vi "Dashboard Main.vi"() -> ()   [LabVIEW 2015]
uses:
  <vilib>/Utility/miscctls.llb/LVRowAndColumnTypeDef.ctl
  <vilib>/event_ctls.llb/eventvkey.ctl
  <vilib>/Rock Robotics/WPI/Dashboard/WPI_DashboardLogging Global.vi
  <vilib>/Rock Robotics/Network Tables/NT Read Numeric Array.vi
  <vilib>/Rock Robotics/Network Tables/NT Read Boolean.vi
  <vilib>/Rock Robotics/Network Tables/NT Write Boolean.vi
  <vilib>/Utility/config.llb/Write Key (String).vi
  <vilib>/Utility/config.llb/Write Key (I32).vi
  <vilib>/Utility/config.llb/NI_LVConfig.lvlib
panel:
  in  "TCP":refnum<k5>
  in  "Rec Mode":enum32{"Stop", "Record", "Playback"}(radio)
  in  "Vision":u16(ring) items=["Camera Off", "USB Camera SW", "USB Camera HW", "IP Camera"]
  out "Camera IP":string
  out "Image Message":string="Timeout in Camera Communications"
  in  "Dashboard Tab":T1(tab)
  in  "Select Auto":string(combo)
  out "NT Connection":bool
  in  "Camera Settings":T2={"Frame Rate"=30, "Compression"=30, "Size"=1} {"Frame Rate" scale=1.0..30.0; "Size" items=["640x480", "320x240", "160x120"]}
  out "MotorChart R":cluster{"Numeric":dbl, "Numeric":dbl}(graph)
  out "MotorChart L":T3(graph)
  out "MotorSliders R":cluster{"MotorSlide1":dbl, "MotorSlide2":dbl} {"MotorSlide2" scale=-1.0..1.0 scale format="%#_2e"; "MotorSlide1" scale=-1.0..1.0 scale format="%#_2e"}
  out "MotorSliders L":T4 {"MotorSlide4 2" scale=0.0..14.0 scale format="%#_2e"; "MotorSlide2" scale=-1.0..1.0 scale format="%#_2e"; "MotorSlide1" scale=-1.0..1.0 scale format="%#_2e"}
  out "Gyro":dbl(knob) scale=0.0..360.0
  out "JS1 Z":dbl(slide) scale=-1.0..1.0 scale format="%#_2e"
  out "JS1 Graph":cluster{"X":dbl, "Y":dbl}[](graph)
  out "JS1 Buttons":T5
  out "JS2 Z":dbl(slide) scale=-1.0..1.0 scale format="%#_2e"
  out "JS2 Graph":cluster{"X":dbl, "Y":dbl}[](graph)
  out "JS2 Buttons":T5
  out "Mode":T6(ring)=enum."Auto Disabled"
  in  "DB Camera Config":bool
  out "fps":dbl format="%#.1g"
  out "Mbps":dbl format="%#.1g"
  out "Mbps LED":bool
  in  "DB/String 9":string
  in  "DB/String 8":string
  in  "DB/String 7":string
  in  "DB/String 6":string
  in  "DB/String 5":string
  in  "DB/String 4":string
  in  "DB/String 3":string
  in  "DB/String 2":string
  in  "DB/String 1":string
  in  "DB/String 0":string
  in  "DB/Slider 0":dbl(slide) scale=0.0..5.0
  in  "DB/Slider 1":dbl(slide) scale=0.0..5.0
  in  "DB/Slider 2":dbl(slide) scale=0.0..5.0
  in  "DB/Slider 3":dbl(slide) scale=0.0..5.0
  out "DB/LED 3":bool
  out "DB/LED 2":bool
  out "DB/LED 1":bool
  out "DB/LED 0":bool
  in  "DB/Button 3":bool
  in  "DB/Button 2":bool
  in  "DB/Button 1":bool
  in  "DB/Button 0":bool caption="New Name"
  in  "Lower Shoot On Start of Auto":bool=TRUE
  in  "Auto Mode \nSelector":dbl
  out "?":dbl(slide)=88.0 scale=78.0..98.0
  out "POT Online?":bool
  out "?":dbl(knob)=87.99999517335185 scale=78.0..98.0
  out "True Solid Value":dbl=88.0
  out "POT Sensor":dbl(knob)=88.0000526149156 scale=78.0..98.0
  out "Low Sensor":bool=TRUE
  out "High Sensor":bool=TRUE
  in  "Test Slider":dbl(slide) scale=0.0..100.0 scale format="%#_3g"
  in  "On/Off":bool caption="Solenoid"
  in  "Test Name":u16(ring) items=["Select the test to run..."]
  in  "Test Tree":string(tree)
  in  "Motor":cluster{"Value":dbl, "Enable":bool} {"Value" scale=-1.0..1.0 scale format="%#_3g"}
  out "Progress":T7 {"Test Progress" scale=0.0..100.0}
  in  "Rev/Fwd":cluster{"Forward":bool, "Reverse":bool}
  in  "Test Ring":u16(ring) items=["Monochrome", "Color"]
  out "Cmd Status":string
  in  "Execute Command":bool
  in  "Command Params":string[][](table)
  in  "Command Selection":i32(listbox)
  in  "CheckList":i32(listbox)
  out "Tree":string(tree)
  out "Camera Image":T8(plugin-control)
  out "Background":bool
  # "Left"
  # "Front"
  # "Right"
  # "Battery"
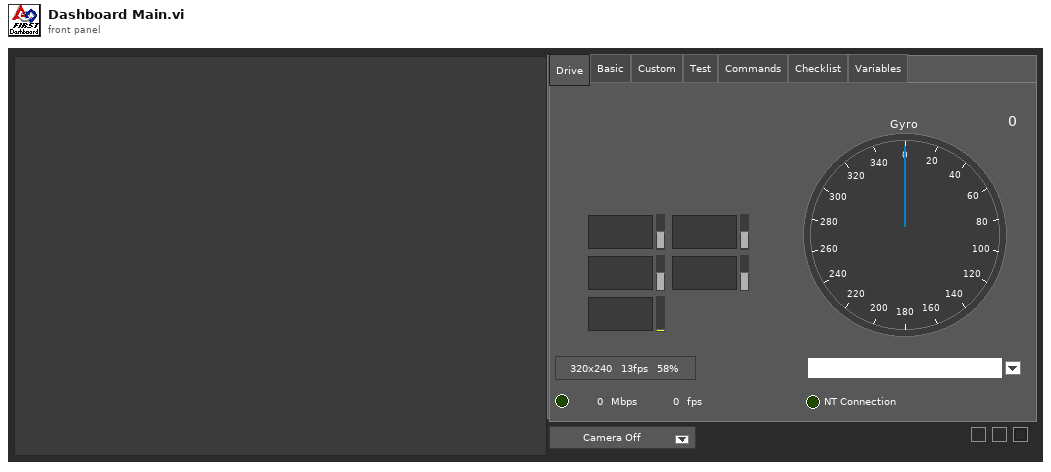
[diagram p1: front panel]
types:
  T1 = enum32{"Drive", "Basic", "Custom", "Test", "Commands", "Checklist", "Variables"}
  T2 = cluster{"Frame Rate":i32, "Compression":i32, "Size":u16}
  T3 = cluster{"Numeric":dbl, "Numeric":dbl, "Battery V":dbl}
  T4 = cluster{"MotorSlide1":dbl, "MotorSlide2":dbl, "MotorSlide4 2":dbl}
  T5 = cluster{bool, bool, bool, bool, bool, bool, bool, bool, bool, bool, bool, bool}
  T6 = enum8{"Tele-Op Disabled", "Tele-Op Enabled", "Auto Disabled", "Auto Enabled", "Test Disabled", "Test Enabled", "Disconnected", "No Code", "E-Stop"}
  T7 = cluster{"Test Progress":u8, "Test Progress Text":string}
  T8 = typedef "IMAQ Image.ctl" = refnum<image>
  T9 = cluster{"IDs":cluster{"RPC field ID":u16, "Unique ID":u16}, "String":string}
  T10 = enum32{"Drive", "Basic", "Custom", "Test", "Checklist", "Variables"}
  T11 = typedef "Image Type" = u32
  T12 = cluster{"Camera Image":refnum<vi>, "Dashboard Tab":refnum<vi>, "Background":refnum<vi>, "Vision":refnum<vi>, "Rec Mode":refnum<vi>, "Test Slider":refnum<vi>, "On/Off ":refnum<vi>, "Test Ring":refnum<vi>, "Rev/Fwd":refnum<vi>, "Test Name":refnum<vi>, "Motor":refnum<vi>, "Progress":refnum<vi>, "CheckList":refnum<vi>, "Tree":refnum<vi>, "Test Tree":refnum<vi>, "Command Params":refnum<vi>, "Command Selection":refnum<vi>, "Execute Command":refnum<vi>, "Cmd Status":refnum<vi>}
  T13 = cluster{"Error Strings":string, "Disable Counts":cluster{u16, u16}, "Rail Faults":cluster{u16, u16, u16}, "Robot IP":string, "DB Mode":u8, "Event Info":cluster{"Name":string, "Type":u8, "Number":u16, "Replay":u8}, "Camera Addr":string}
  T14 = cluster{"Storage":cluster{"Disk Free":u64, "RAM Block":u32, "RAM free":u32}, "CPU Utilization":cluster{"CPU % ISR":sgl, "CPU % Time Crit":sgl, "CPU % Timed Str":sgl, "CPU % High":sgl, "CPU % Above":sgl, "CPU % Normal":sgl, "CPU % Low":sgl}, "CAN":cluster{"% Bus Utilization":sgl, "Bus Off Cnt":u32, "TX_FIFO Full Cnt":u32, "Receive Error Cnt":u8, "Transmit Error Cnt":u8}, "HID":cluster{"HID Outputs":u32, "Rumble Low":u16, "Rumble High":u16}[]}
  T15 = cluster{"Status bits":cluster{"Test Mode":bool, "Autonomous":bool, "Enabled":bool, "Code Start":bool, "Brownout":bool, "Reserved 2":bool, "Reserved 3":bool, "E-Stop":bool}, "Code Trace":cluster{"Disabled":bool, "TeleOp":bool, "Auto":bool, "Test":bool}, "Controller Type":enum16{"unknown", "cRIO", "roboRio"}, "Code?":enum16{"unknown", "noCode", "code"}, "Battery V":dbl}
  T16 = cluster{"Control Bits":cluster{"TestMode":bool, "Autonomous":bool, "Enabled":bool, "FMS Present":bool, bool, bool, bool, "E-Stop":bool}, "Team Station ":u8, "Countdown":sgl, "Joystick Values":cluster{"Axes":dbl[], "Buttons":bool[], "POVs":i16[]}[]}
  T17 = cluster{"Axes":dbl[], "Buttons":bool[], "POVs":i16[]}[]
  T18 = cluster{"Axes":dbl[], "Buttons":bool[], "POVs":i16[]}
  T19 = cluster{"Buttons[0]":bool, "Buttons[1]":bool, "Buttons[2]":bool, "Buttons[3]":bool, "Buttons[4]":bool, "Buttons[5]":bool, "Buttons[6]":bool, "Buttons[7]":bool, "Buttons[8]":bool, "Buttons[9]":bool, "Buttons[10]":bool, "Buttons[11]":bool}
  T20 = typedef "NI_LVConfig.lvlib/Config Data RefNum.ctl" = refnum<k1>
  T21 = cluster{"Operation":enum16{"Update", "Clear"}, "Color Box":u32}[]
  T22 = typedef "eventvkey.ctl" = enum16{"ASCII", "Enter", "Return", "Shift", "Ctrl", "Alt", "Cmd", "Opt", "Caps", "NumLock", "Clear", "Break", "Up", "Down", "Left", "Right", "Insert", "Delete", "Home", "End", "PageUp", "PageDown", "Escape", "Help", "Pause", "ScrollLock", "F1", "F2", "F3", "F4", "F5", "F6", "F7", "F8", "F9", "F10", "F11", "F12", "F13", "F14", "F15", "F16", "F17", "F18", "F19", "F20", "F21", "F22", "F23", "F24", "Play", "VolumeUp", "VolumeDown", "Mute", "Two Byte Char"}
  T23 = cluster{"Image Size":bool, "Image Type":bool, "Pixel Value":bool, "ROI Information":bool, "Zoom Factor":bool}
  T24 = enum8{"Enabled", "Disabled", "Disabled and Grayed Out"}
  T25 = cluster{"Operation":enum16{"Update", "Clear"}, "Color Box":u32}
  T26 = typedef "LVRowAndColumnTypeDef.ctl" = cluster{"Row":i32, "Column":i32}
  T27 = cluster{"Shift":bool, "Ctrl":bool, "Alt":bool, "Cmd":bool, "Opt":bool}
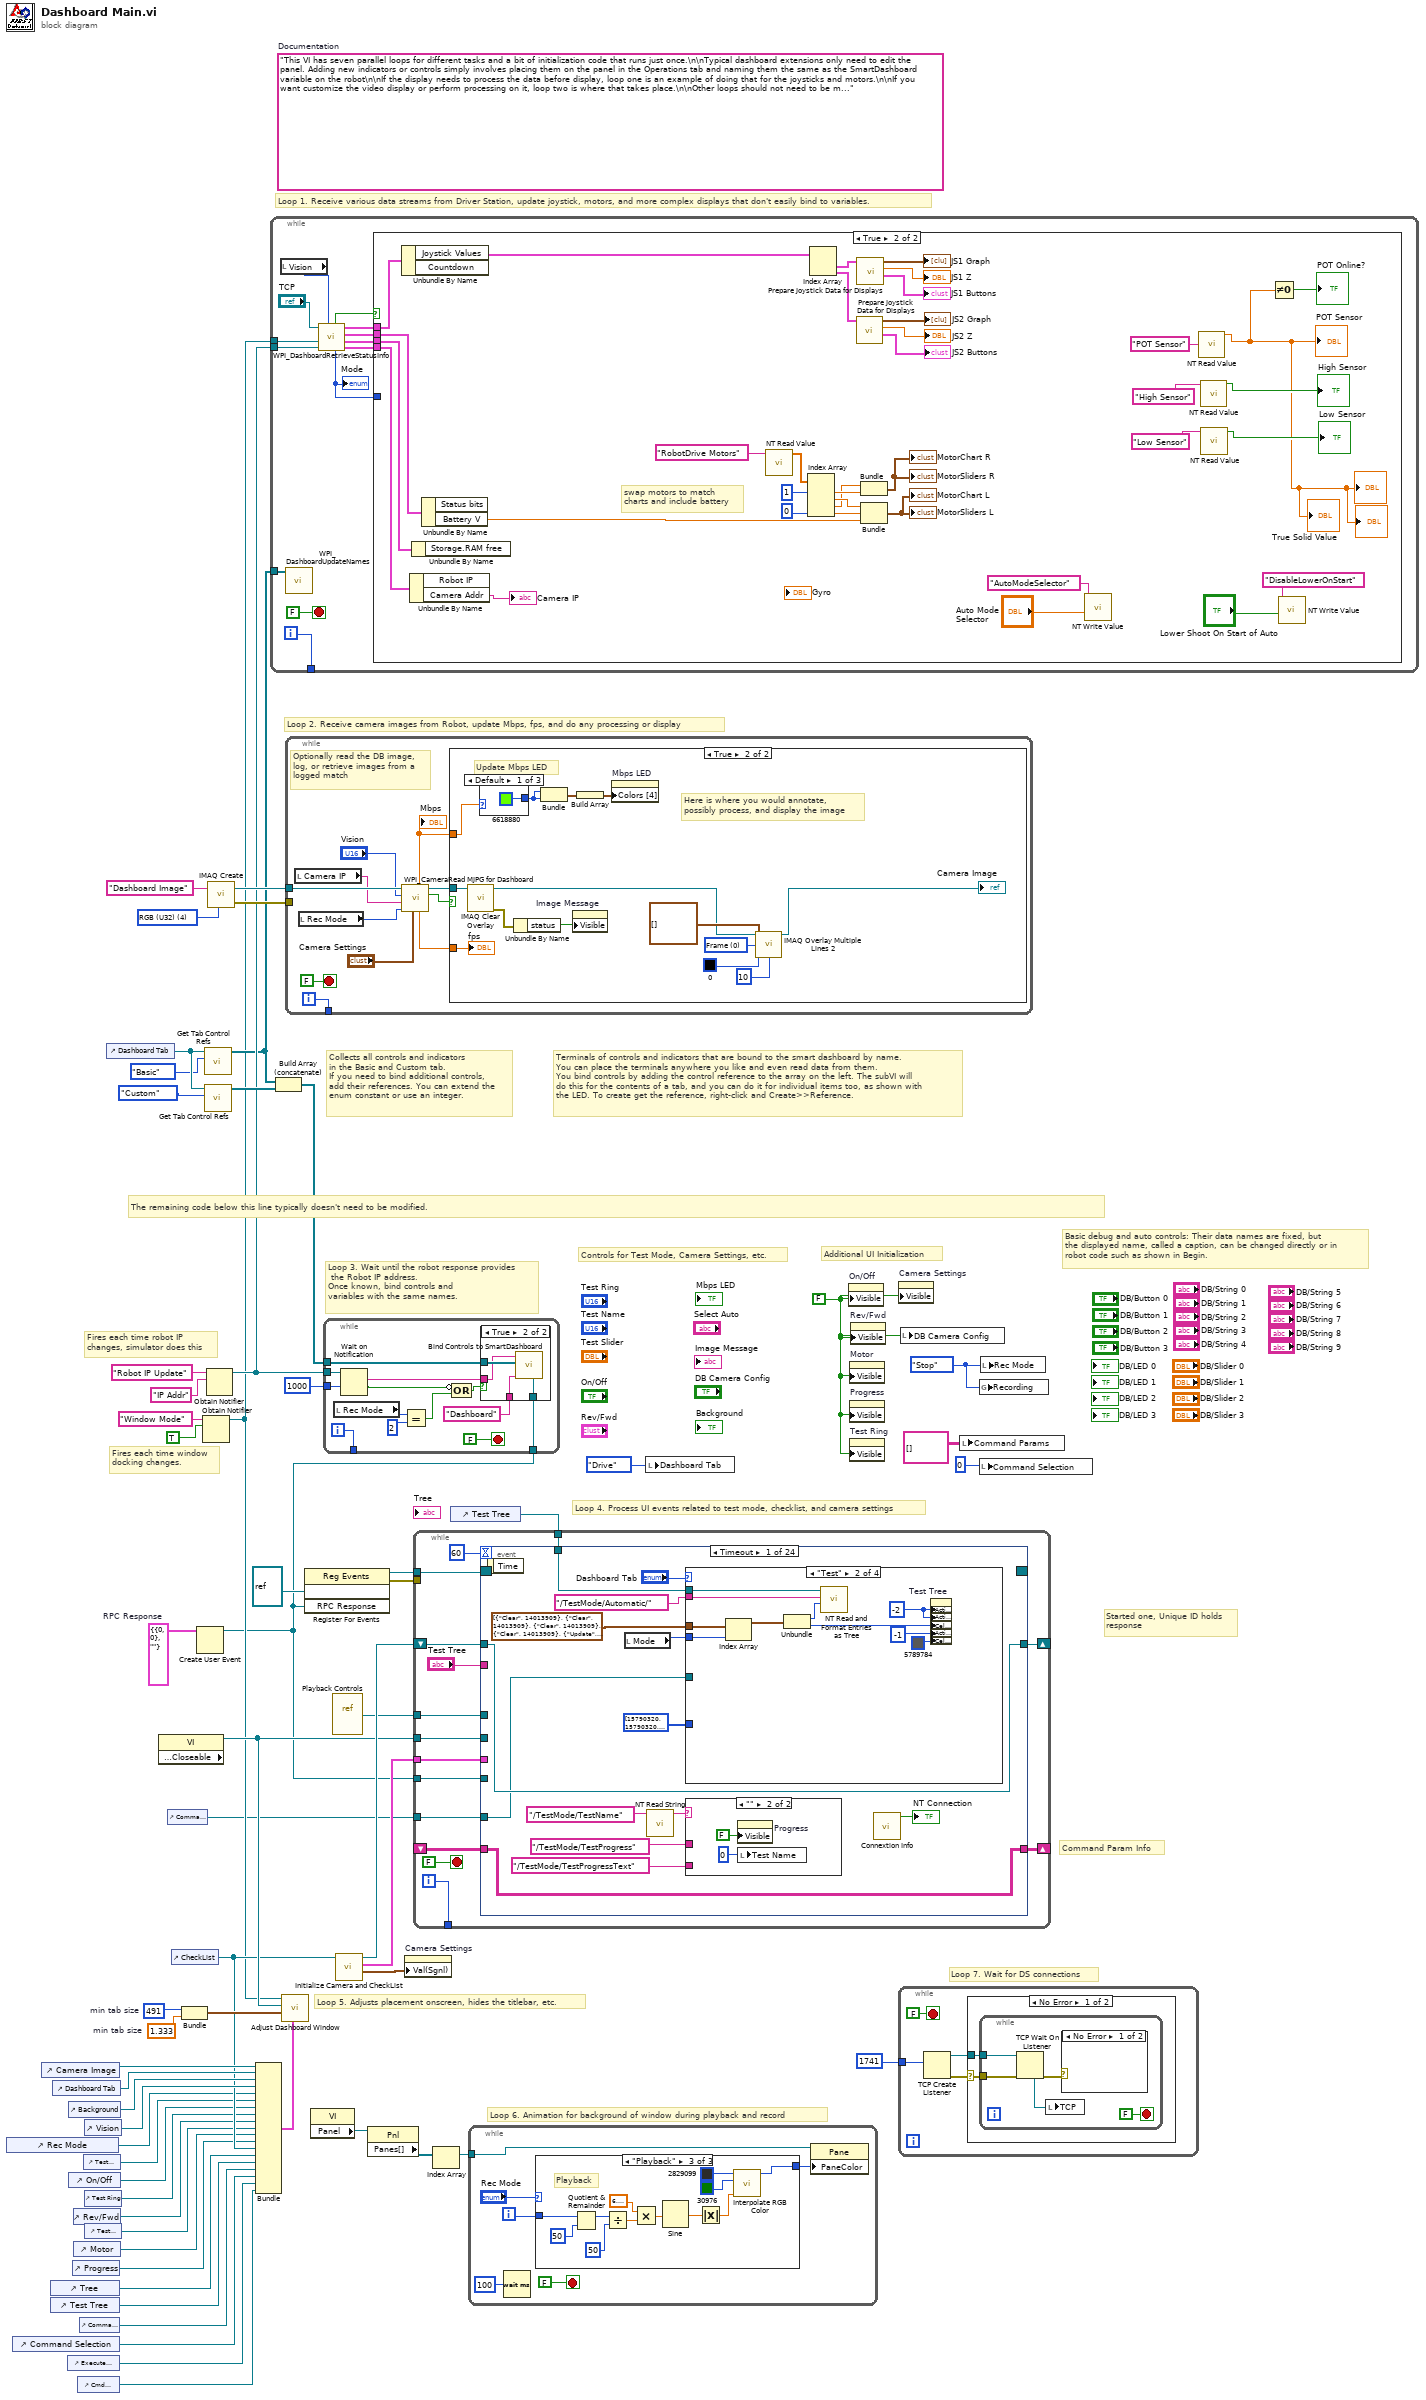
[diagram p0: block diagram]
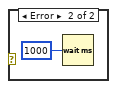
[diagram p2: hidden frame]
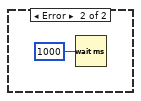
[diagram p3: hidden frame]
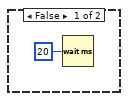
[diagram p4: hidden frame]
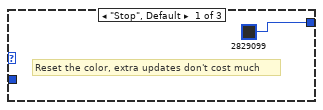
[diagram p5: hidden frame]
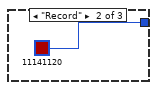
[diagram p6: hidden frame]
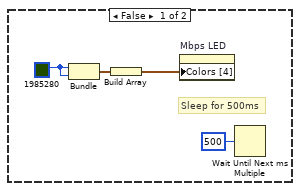
[diagram p8: hidden frame]
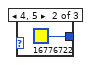
[diagram p9: hidden frame]
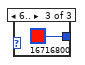
[diagram p10: hidden frame]
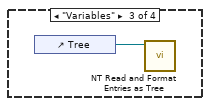
[diagram p12: hidden frame]
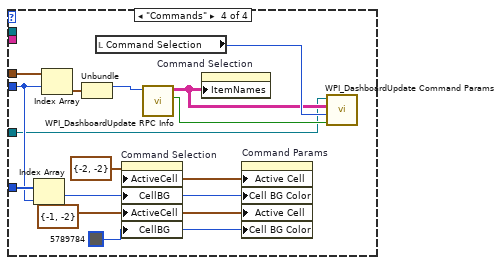
[diagram p13: hidden frame]
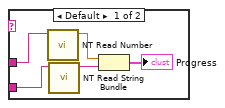
[diagram p14: hidden frame]
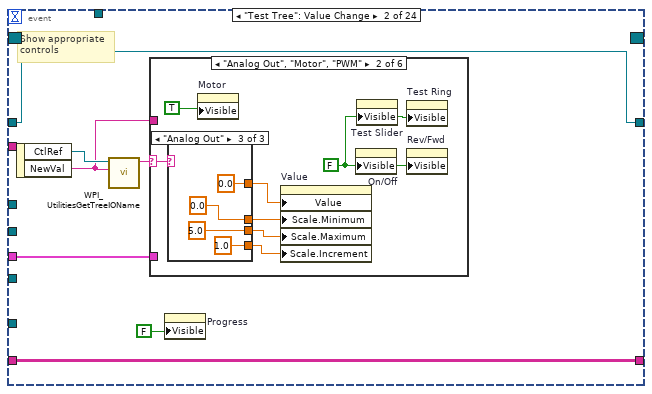
[diagram p15: hidden frame]
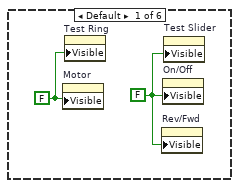
[diagram p16: hidden frame]
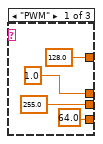
[diagram p17: hidden frame]
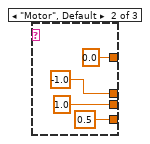
[diagram p18: hidden frame]
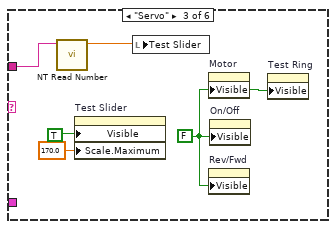
[diagram p19: hidden frame]
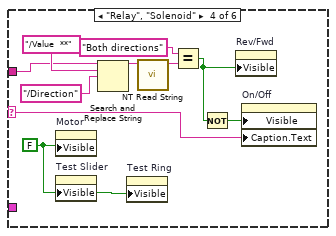
[diagram p20: hidden frame]
diagram:
  w7 = T9 {"IDs"={"RPC field ID"=0, "Unique ID"=0}, "String"=""}  # RPC Response
  w33 = 491  # min tab size
  w32 = 1.333  # min tab size
  w41 = enum32{"Stop", "Record", "Playback"}."Stop" ("Rec Mode")
  w15 = FALSE ("Visible")
  (unwired) "This VI has seven parallel loops for different tasks and a bit of initialization code that runs just once.\n\nTypical dashboard extensions only need to edit the panel. Adding new indicators or controls simply involves placing them on the panel in the Operations tab and naming them the same as the SmartDashboard variable on the robot\n\nIf the display needs to process the data before display, loop one is an example of doing that for the joysticks and motors.\n\nIf you want customize the video display or perform processing on it, loop two is where that takes place.\n\nOther loops should not need to be modified. They are pretty standard, and document the task they perform."  # Documentation
  w61 = T11 4 items=["Grayscale (U8)", "Grayscale (I16)", "Grayscale (SGL)", "Complex (CSG)", "RGB (U32)", "HSL (U32)", "RGB (U64)"] ("Image Type")
  # "Command Param Info"
  # "Started one, Unique ID holds\nresponse"
  # "Loop 7. Wait for DS connections"
  # "Basic debug and auto controls: Their data names are fixed, but\nthe displayed name, called a caption, can be changed directly or in\nrobot code such as shown in Begin."
  # "Controls for Test Mode, Camera Settings, etc."
  # "Additional UI Initialization"
  # "Loop 6. Animation for background of window during playback and record"
  # "Fires each time robot IP\nchanges, simulator does this"
  # "Fires each time window\ndocking changes."
  # "Collects all controls and indicators\nin the Basic and Custom tab.\nIf you need to bind additional controls,\nadd their references. You can extend the\nenum constant or use an integer."
  # "The remaining code below this line typically doesn't need to be modified."
  # "Loop 4. Process UI events related to test mode, checklist, and camera settings"
  # "Terminals of controls and indicators that are bound to the smart dashboard by name.\nYou can place the terminals anywhere you like and even read data from them.\nYou bind controls by adding the control reference to the array on the left. The subVI will\ndo this for the contents of a tab, and you can do it for individual items too, as shown with\nthe LED. To create get the reference, right-click and Create>>Reference."
  # "Loop 3. Wait until the robot response provides\n the Robot IP address.\nOnce known, bind controls and\nvariables with the same names."
  # "Loop 5. Adjusts placement onscreen, hides the titlebar, etc."
  # "Loop 1. Receive various data streams from Driver Station, update joystick, motors, and more complex displays that don't easily bind to variables."
  # "Loop 2. Receive camera images from Robot, update Mbps, fps, and do any processing or display"
  n1 = control-ref of="Rec Mode"() -> (w21:refnum<vi>)
  n2 = control-ref of="Command Selection"() -> (w6:refnum<vi>)
  n3 = control-ref of="Camera Image"() -> (w36:refnum<vi>)
  n4 = control-ref of="Tree"() -> (w25:refnum<vi>)
  n5 = control-ref of="Test Tree"() -> (w24:refnum<vi>)
  n6 = control-ref of="Dashboard Tab"() -> (w35:refnum<vi>)
  n7 = control-ref of="Execute Command"() -> (w8:refnum<vi>)
  n8 = control-ref of="Background"() -> (w30:refnum<vi>)
  n9 = control-ref of="On/Off"() -> (w19:refnum<vi>)
  n10 = control-ref of="Progress"() -> (w16:refnum<vi>)
  n11 = control-ref of="Rev/Fwd"() -> (w17:refnum<vi>)
  n12 = control-ref of="Motor"() -> (w22:refnum<vi>)
  n13 = control-ref of="Cmd Status"() -> (w2:refnum<vi>)
  n14 = control-ref of="Command Params"() -> (w9:refnum<vi>)
  n15 = control-ref of="Test Slider"() -> (w20:refnum<vi>)
  n16 = control-ref of="Vision"() -> (w34:refnum<vi>)
  n17 = control-ref of="Test Ring"() -> (w18:refnum<vi>)
  n18 = control-ref of="Test Name"() -> (w23:refnum<vi>)
  n19 = control-ref of="Dashboard Tab"() -> (w39:refnum<vi>)
  n20 = property class="VI" props=["Front Panel.Closeable"]() -> (reference out=w40:refnum<vi>)  [unwired: 2 in, 2 out]
  n21 = control-ref of="Command Params"() -> (w1:refnum<vi>)
  n22 = control-ref of="CheckList"() -> (w26:refnum<vi>)
  n23 = Bundle("min tab size"=w33, "min tab size"=w32) -> (w31:cluster{"min tab size":i32, "min tab size":dbl})  [unwired: 1 in]
  n24 = Create User Event(user event datatype=w7) -> (user event=w3:refnum<user-event>)  [unwired: 1 in, 1 out]
  n25 = Obtain Notifier(name (unnamed)="Window Mode", notification data type=TRUE) -> (notifier out=w12:refnum<notifier>)  [unwired: 2 in, 2 out]
  n26 = call <vilib>:"Get Tab Control Refs.vi"("Page Index"=T10."Basic" ("Dashboard Tab"), "TabControl in"=w39) -> ("ControlsOnPage"=w13:refnum<vi>[])  [unwired: 9 in]
  n27 = call <vilib>:"Get Tab Control Refs.vi"("Page Index"=T10."Custom" ("Dashboard Tab"), "TabControl in"=w39) -> ("ControlsOnPage"=w38:refnum<vi>[])  [unwired: 9 in]
  n28 = Obtain Notifier(name (unnamed)="Robot IP Update", notification data type="IP Addr" ("name (unnamed)")) -> (notifier out=w14:refnum<notifier>)  [unwired: 2 in, 2 out]
  n29 = call "IMAQ Create"("Image Name"="Dashboard Image", "Image Type"=w61) -> ("New Image"=w59:T8, "error out"=w58:errorcluster)  [unwired: 2 in, 1 out]
  n30 = Bundle("Camera Image"=w36, "Dashboard Tab"=w35, "Background"=w30, "Vision"=w34, "Rec Mode"=w21, "Test Slider"=w20, "On/Off"=w19, "Test Ring"=w18, "Rev/Fwd"=w17, "Test Name"=w23, "Motor"=w22, "Progress"=w16, "CheckList"=w26, "Tree"=w25, "Test Tree"=w24, "Command Params"=w9, "Command Selection"=w6, "Execute Command"=w8, "Cmd Status"=w2) -> (w27:T12)  [unwired: 1 in]
  n31 = while {
    tunnel: [w73] -> _
    tunnel: w14 -> [w67]
    tunnel: w13 -> [w66]
    tunnel: w12 -> [w62]
    i -> [w73]
    stop <- FALSE stop-if-true
    n32 = local read "Vision"() -> (w64:u16)
    n33 = call <vilib>:"WPI_DashboardUpdateNames.vi"("Controls on Tab"=w66) -> ()  [unwired: 11 in]
    n34 = call <vilib>:"WPI_DashboardRetrieveStatusInfo.vi"("Vision"=w64, "Binding Refnum"=w67, "Window Mode Notifier"=w62, "TCP Cnx"="TCP") -> ("Power and Errors"=w68:T13, "Robot Metrics"=w71:T14, "Status Info"=w72:T15, "Control Info"=w69:T16, "Robot Mode"=w65:T6, "Process?"=w70:bool)  [unwired: 2 in]
    "Mode" <- w65
    n35 = case shown="True" w70 {
      tunnel: w72 -> [_ w111]
      tunnel: w71 -> [_ w110]
      tunnel: w69 -> [_ w109]
      tunnel: w68 -> [_ w108]
      tunnel: w65 -> [_ _]
      frame False {
        n36 = Wait (ms)(milliseconds to wait=u32 20) -> ()  [unwired: 1 out]
      }
      frame True {
        # "swap motors to match\ncharts and include battery"
        n37 = Unbundle By Name(w109) -> ("Joystick Values"=w98:T17)  [unwired: 1 out]
        n38 = Unbundle By Name(w108) -> ("Camera Addr"=→"Camera IP":string)  [unwired: 1 out]
        n39 = Unbundle By Name(w110) -> ()  [unwired: 1 out]
        n40 = Unbundle By Name(w111) -> ("Battery V"=w99:dbl)  [unwired: 1 out]
        n41 = call-poly <vilib>:"NT Read Value.vi"("Name"="RobotDrive Motors") -> ("Numeric Array"=w87:dbl[])  [unwired: 9 in, 1 out]
        n42 = Index Array(array=w87, index #1=1, index #4=0) -> (element #1=w103:dbl, element #2=w104:dbl, element #3=w102:dbl, element #4=w107:dbl)  [unwired: 2 in]
        n43 = Index Array(array=w98) -> (element #1=w97:T18, element #2=w92:T18)  [unwired: 2 in]
        n44 = call "Prepare Joystick Data for Displays.vi"("Joystick Values"=w92) -> ("Buttons"=→"JS2 Buttons":T19, "Z Axis"=→"JS2 Z":dbl, "Cartesian Data"=→"JS2 Graph":cluster{"X axis":dbl, "X axis":dbl}[])  [unwired: 8 in]
        n45 = call "Prepare Joystick Data for Displays.vi"("Joystick Values"=w97) -> ("Buttons"=→"JS1 Buttons":T19, "Z Axis"=→"JS1 Z":dbl, "Cartesian Data"=→"JS1 Graph":cluster{"X axis":dbl, "X axis":dbl}[])  [unwired: 8 in]
        n46 = Bundle("Numeric"=w102, "Numeric"=w103) -> (→"MotorChart R" →"MotorSliders R":cluster{"Numeric":dbl, "Numeric":dbl})  [unwired: 1 in]
        n47 = Bundle("Numeric"=w104, "Numeric"=w107, "Battery V"=w99) -> (→"MotorChart L" →"MotorSliders L":T3)  [unwired: 1 in]
        n48 = call-poly <vilib>:"NT Write Value.vi"("Numeric"="Auto Mode \nSelector", "Name"="AutoModeSelector") -> ()  [unwired: 9 in, 1 out]
        n49 = call-poly <vilib>:"NT Read Value.vi"("Name"="POT Sensor") -> ("Numeric"=w76:dbl)  [unwired: 9 in, 1 out]
        "POT Sensor" <- w76
        "True Solid Value" <- w76
        "?" <- w76
        "?" <- w76
        n50 = call-poly <vilib>:"NT Read Value.vi"("Name"="High Sensor") -> ("Boolean"=→"High Sensor":bool)  [unwired: 9 in, 1 out]
        n51 = call-poly <vilib>:"NT Read Value.vi"("Name"="Low Sensor") -> ("Boolean"=→"Low Sensor":bool)  [unwired: 9 in, 1 out]
        n52 = Not Equal To 0?(x=w76) -> (x != 0?=→"POT Online?":bool)
        n53 = call-poly <vilib>:"NT Write Value.vi"("Boolean"="Lower Shoot On Start of Auto", "Name"="DisableLowerOnStart") -> ()  [unwired: 9 in, 1 out]
      }
    }
  }
  n54 = Build Array (concatenate)(w13, w38) -> (w37:refnum<vi>[])
  n55 = call "Adjust Dashboard Window.vi"("Sizing Refnums"=w27, "Size Constraints"=w31, "VI"=w40, "WIn Mode"=w12) -> ()  [unwired: 8 in]
  n56 = while {
    tunnel: w59 -> [w120]
    tunnel: w58 -> [_]
    tunnel: [w121] -> _
    i -> [w121]
    stop <- FALSE stop-if-true
    # "Optionally read the DB image,\nlog, or retrieve images from a\nlogged match"
    n57 = local read "Camera IP"() -> (w112:string)
    n58 = local read "Rec Mode"() -> (w115:enum32{"Stop", "Record", "Playback"})
    n59 = call <vilib>:"WPI_CameraRead MJPG for Dashboard.vi"("Camera Settings"="Camera Settings", "Rec Mode"=w115, "Camera IP"=w112, "Camera Mode"="Vision", "Refnum in"=w120) -> ("Active"=w118:bool, "Refnum out"=w119:T8, "FPS"=w117:dbl, "Bandwidth (Mbps)"=w113:dbl)  [unwired: 3 in]
    "Mbps" <- w113
    n60 = case shown="True" w118 {
      tunnel: w119 -> [_ w135]
      tunnel: w113 -> [_ w134]
      tunnel: w117 -> [_ w133]
      frame False {
        w123 = u32 1985280 ("Color Box")
        # "Sleep for 500ms"
        n61 = Bundle("Color Box"=w123, "Color Box"=w123) -> (w125:cluster{"Color Box":u32, "Color Box":u32})  [unwired: 1 out]
        n62 = Build Array(w125) -> (w124:cluster{"Color Box":u32, "Color Box":u32}[])
        n63 = property on="Mbps LED" class="Bool (strict)"("Colors [4]"=w124) -> ()  [unwired: 2 in, 2 out]
        n64 = Wait Until Next ms Multiple(millisecond multiple=u32 500) -> ()  [unwired: 1 out]
      }
      frame True {
        w132 = u32 0 items=["Frame", "Fill"] ("Drawing Mode (Frame)")
        # "Here is where you would annotate,\npossibly process, and display the image"
        # "Update Mbps LED"
        n65 = call "IMAQ Clear Overlay"("Image"=w135) -> ("error out"=w139:errorcluster, "Image Out"=w129:T8)  [unwired: 2 in, 7 out]
        n66 = case shown="Default" w134 {
          tunnel: [u32 6618880 ("Color Box") u32 16776722 ("Color Box") u32 16716800 ("Color Box")] -> w136
          frame Default {
          }
          frame 4, 5 {
          }
          frame 6.. {
          }
        }
        n67 = Unbundle By Name(w139) -> ("status"=w140:bool)
        n68 = Bundle("Color Box"=w136, "Color Box"=w136) -> (w138:cluster{"Color Box":u32, "Color Box":u32})  [unwired: 1 out]
        n69 = property on="Image Message" class="Str"("Visible"=w140) -> ()  [unwired: 2 in, 2 out]
        n70 = Build Array(w138) -> (w137:cluster{"Color Box":u32, "Color Box":u32}[])
        n71 = property on="Mbps LED" class="Bool (strict)"("Colors [4]"=w137) -> ()  [unwired: 2 in, 2 out]
        n72 = call "IMAQ Overlay Multiple Lines 2"("Image"=w129, "Line End Points"=cluster{"X":dbl, "Y":dbl}[] [], "Drawing Mode (Frame)"=w132, "Color"=u32 0, "Width"=u32 10) -> ("Image Out"=→"Camera Image":T8)  [unwired: 9 in, 1 out]
        "fps" <- w133
      }
    }
  }
  n73 = register-events(refnum<vi> refnum, w3) -> (reference out=w45:refnum<event-registration>, error out=w44:errorcluster)  [unwired: 2 in]
  n74 = property class="VI"() -> ("Panel"=w48:refnum<vi>)  [unwired: 2 in, 2 out]
  n75 = while {
    tunnel: w37 -> [w156]
    tunnel: w14 -> [w154]
    tunnel: [w152] -> _
    tunnel: u32 1000 ("milliseconds to wait") -> [w151]
    tunnel: w3 -> [w144]
    i -> [w152]
    stop <- FALSE stop-if-true
    n76 = local read "Rec Mode"() -> (w147:enum32{"Stop", "Record", "Playback"})
    n77 = Wait on Notification(notifier=w154, timeout in ms (-1)=w151) -> (notification=w153:string, timed out?=w149:bool)  [unwired: 2 in, 2 out]
    n78 = Equal?(x=w147, y=u16 2 ("Rec Mode")) -> (x = y?=w148:bool)
    n79 = Compound Arithmetic op=OR(invert w149, w148) -> (w150:bool)
    n80 = case shown="True" w150 {
      tunnel: w156 -> [_ w160]
      tunnel: w153 -> [_ w159]
      tunnel: "Dashboard" -> [_ w158]
      tunnel: w144 -> [_ w157]
      frame False {
      }
      frame True {
        n81 = call <vilib>:"Bind Controls to SmartDashboard.vi"("RPC ref"=w157, "Client Name"=w158, "Bound Control Refs"=w160, "Server IP Address"=w159) -> ()  [unwired: 8 in]
      }
    }
  }
  n82 = vi-ref "Playback Controls.vi"() -> (w46:refnum<vi>)
  n83 = call "Initialize Camera and CheckList.vi"("ListBox in"=w26) -> ("Cluster"=w52:cluster{"value":i32, "value":i32, "index":i32}, "Array"=w53:cluster{string[]}[], "File Refnum"=w51:T20)  [unwired: 8 in]
  n84 = property class="Pnl"(reference=w48) -> ("Panes[]"=w49:refnum<vi>[])  [unwired: 1 in, 2 out]
  n85 = property on="Camera Settings" class="Clust (strict)"("Val(Sgnl)"=w52) -> ()  [unwired: 2 in, 2 out]
  n86 = Index Array(array=w49) -> (element=w47:refnum<vi>)  [unwired: 1 in]
  n87 = control-ref of="Test Tree"() -> (w50:refnum<vi>)
  n88 = while {
    tunnel: w53 -> [w172]
    shift-right: [w171] -> _
    shift-left: w51 -> [w170]
    tunnel: [w169] -> _
    tunnel: w50 -> [w168]
    tunnel: w46 -> [w167]
    tunnel: w45 -> [w166]
    tunnel: w44 -> [_]
    tunnel: w40 -> [w165]
    tunnel: w3 -> [w164]
    tunnel: w1 -> [w163]
    shift-right: [w162] -> _
    shift-left: _ -> [w161]
    i -> [w169]
    stop <- FALSE stop-if-true
    n89 = event shown="[0] Timeout" {
      selector: w166 -> [_ _ _ _ _ _ _ _ _ _ _ _ _ _ _ _ _ _ _ _ _ _ _ _]
      dyn-events: [_ _ _ _ _ _ _ _ _ _ _ _ _ _ _ _ _ _ w481 _ _ _ _ _] -> _
      timeout: u32 60 ("milliseconds to wait") -> [_ _ _ _ _ _ _ _ _ _ _ _ _ _ _ _ _ _ _ _ _ _ _ _]
      tunnel: w168 -> [w185 _ _ _ _ _ _ _ _ _ _ _ _ _ _ _ _ _ _ _ _ _ _ _]
      tunnel: "Test Tree" -> [_ _ _ _ _ _ _ _ _ _ _ _ _ w444 w453 w456 w461 w470 _ _ _ _ _ _]
      tunnel: w172 -> [_ w223 _ _ _ _ _ _ _ _ _ w406 w437 _ _ _ _ _ _ _ _ _ _ _]
      tunnel: [w182 w222 w326 w332 w342 w346 w352 w364 w372 w378 w391 w405 w430 w443 w451 w455 w460 w469 w483 w499 w501 w509 w520 w525] -> w171
      tunnel: w170 -> [w182 w222 w326 w332 w342 w346 w352 w364 w372 w378 w391 w404 w430 w443 w451 w455 w460 w469 w483 w499 w501 w509 w520 w525]
      tunnel: w167 -> [_ _ _ _ _ _ _ _ _ _ _ _ _ _ _ _ _ _ w484 _ w504 _ _ _]
      tunnel: w165 -> [_ _ _ _ _ _ _ _ _ _ _ _ _ _ _ _ _ _ w479 _ _ _ _ _]
      tunnel: w164 -> [_ _ _ _ _ _ _ _ _ _ _ _ _ _ _ _ _ _ w475 _ _ _ _ _]
      tunnel: w163 -> [w177 _ _ _ _ _ w350 _ _ _ _ _ _ _ _ _ _ _ _ _ _ _ _ _]
      tunnel: [w176 w221 w325 w331 w341 w347 w348 w358 w369 w377 w390 w403 w429 w442 w450 w454 w459 w468 w474 w497 w500 w505 w513 w526] -> w162
      tunnel: w161 -> [w176 w221 w325 w331 w341 w347 w348 _ _ w377 w390 w403 w429 w442 w450 w454 w459 w468 w474 w497 w500 w505 w513 w526]
      event Timeout {
        n90 = event-data() -> ()  [unwired: 1 in, 1 out]
        n91 = local read "Mode"() -> (w179:T6)
        n92 = call <vilib>:"NT Read String.vi"("Name"="/TestMode/TestName") -> ("String"=w188:string)  [unwired: 9 in, 1 out]
        n93 = case shown="\"Test\"" "Dashboard Tab" {
          tunnel: w185 -> [_ w199 _ _]
          tunnel: "/TestMode/Automatic/" ("Name Pattern") -> [_ w198 _ _]
          tunnel: T21 [{"Operation"=enum."Clear", "Color Box"=14013909}, {"Operation"=enum."Clear", "Color Box"=14013909}, {"Operation"=enum."Clear", "Color Box"=14013909}, {"Operation"=enum."Clear", "Color Box"=14013909}, {"Operation"=enum."Update", "Color Box"=14013909}, {"Operation"=enum."Update", "Color Box"=16777215}, {"Operation"=enum."Clear", "Color Box"=14013909}, {"Operation"=enum."Clear", "Color Box"=14013909}, {"Operation"=enum."Clear", "Color Box"=14013909}] -> [_ w191 _ w208]
          tunnel: w179 -> [_ w190 _ w207]
          tunnel: u32[] [15790320, 15790320, 15790320, 15790320, 16777215, 16777215, 15790320, 15790320, 15790320] -> [_ _ _ w213]
          tunnel: w177 -> [_ _ _ w201]
          frame "Custom", Default {
          }
          frame "Test" {
            w197 = -2 ("Active Item:Row Number")
            n94 = Index Array(array=w191, index=w190) -> (element=w192:T25)
            n95 = Unbundle(w192) -> ("Operation"=w193:enum16{"Update", "Clear"}, "Color Box"=w194:u32)
            n96 = call <vilib>:"NT Read and Format Entries as Tree.vi"("Operation"=w193, "Name Pattern"=w198, "Tree Refnum"=w199) -> ()  [unwired: 7 in, 2 out]
            n97 = property on="Test Tree" class="Tree (strict)"("Active Item Row Number"=w197, "ActiveColNum"=w197, "CellBG"=w194, "Active Item Row Number"=-1 ("Active Item:Row Number"), "CellBG"=u32 5789784 ("Color Box")) -> ()  [unwired: 2 in, 2 out]
          }
          frame "Variables" {
            n98 = control-ref of="Tree"() -> (w200:refnum<vi>)
            n99 = call <vilib>:"NT Read and Format Entries as Tree.vi"("Tree Refnum"=w200) -> ()  [unwired: 9 in, 2 out]
          }
          frame "Commands" {
            w209 = u32 5789784 ("Color Box")
            w210 = T26 {"Row"=-1, "Column"=-2} ("Active Cell:Active Cell")
            w212 = T26 {"Row"=-2, "Column"=-2} ("Active Cell:Active Cell")
            n100 = Index Array(array=w213, index=w207) -> (element=w211:u32)
            n101 = Index Array(array=w208, index=w207) -> (element=w206:T25)
            n102 = Unbundle(w206) -> ("Operation"=w205:enum16{"Update", "Clear"})  [unwired: 1 out]
            n103 = local read "Command Selection"() -> (w204:i32)
            n104 = property on="Command Selection" class="MCListbox (strict)"("ActiveCell"=w212, "CellBG"=w211, "ActiveCell"=w210, "CellBG"=w209) -> ()  [unwired: 2 in, 2 out]
            n105 = call <vilib>:"WPI_DashboardUpdate RPC Info.vi"("Operation"=w205) -> ("update"=w203:bool, "commands"=w202:string[][])  [unwired: 9 in]
            n106 = property on="Command Selection" class="MCListbox (strict)"("ItemNames"=w202) -> ()  [unwired: 2 in, 2 out]
            n107 = property on="Command Params" class="Tbl (strict)"("Active Cell"=w212, "Cell BG Color"=w211, "Active Cell"=w210, "Cell BG Color"=w209) -> ()  [unwired: 2 in, 2 out]
            n108 = call <vilib>:"WPI_DashboardUpdate Command Params.vi"("Update"=w203, "NewVal"=w204, "Commands"=w202, "Param Tbl"=w201) -> ()  [unwired: 7 in, 1 out]
          }
        }
        n109 = case shown="\"\"" w188 {
          tunnel: "/TestMode/TestProgress" ("Name") -> [w215 _]
          tunnel: "/TestMode/TestProgressText" ("Name") -> [w214 _]
          frame Default {
            n110 = call <vilib>:"NT Read Number.vi"("Name"=w215) -> ("Numeric"=w216:dbl)  [unwired: 9 in, 1 out]
            n111 = call <vilib>:"NT Read String.vi"("Name"=w214) -> ("String"=w217:string)  [unwired: 9 in, 1 out]
            n112 = Bundle("Numeric"=w216, "String"=w217) -> (→"Progress":cluster{"Numeric":dbl, "String":string})  [unwired: 1 in]
          }
          frame "" {
            n113 = property on="Progress" class="Clust (strict)"("Visible"=FALSE) -> ()  [unwired: 2 in, 2 out]
            n114 = local write "Test Name"(u16 0) -> ()
          }
        }
        n115 = call <vilib>:"Connextion Info.vi"() -> ("Connected"=→"NT Connection":bool)  [unwired: 10 in, 1 out]
      }
      event "Test Tree": Value Change {
        # "Show appropriate\ncontrols"
        n116 = event-data() -> ("CtlRef"=w226:refnum<vi>, "NewVal"=w224:string)  [unwired: 1 in]
        n117 = call <vilib>:"WPI_UtilitiesGetTreeIOName.vi"("NewVal"=w224, "TreeControl in"=w226) -> ("I/O Name"=w227:string)  [unwired: 9 in]
        n118 = case shown="\"Analog Out\", \"Motor\", \"PWM\"" w227 {
          selector: w227 -> [_ w234 _ w256 w265 _]
          tunnel: w224 -> [_ _ w253 w255 _ w272]
          tunnel: w223 -> [_ _ _ _ _ w271]
          frame Default {
            w229 = FALSE ("Visible")
            w228 = FALSE ("Visible")
            n119 = property on="Motor" class="Clust (strict)"("Visible"=w228) -> ()  [unwired: 2 in, 2 out]
            n120 = property on="Test Ring" class="Ring (strict)"("Visible"=w228) -> ()  [unwired: 2 in, 2 out]
            n121 = property on="Rev/Fwd" class="Clust (strict)"("Visible"=w229) -> ()  [unwired: 2 in, 2 out]
            n122 = property on="On/Off" class="Bool (strict)"("Visible"=w229) -> ()  [unwired: 2 in, 2 out]
            n123 = property on="Test Slider" class="Slide (strict)"("Visible"=w229) -> ()  [unwired: 2 in, 2 out]
          }
          frame "Analog Out", "Motor", "PWM" {
            w235 = FALSE ("Visible")
            n124 = case shown="\"Analog Out\"" w234 {
              tunnel: [1.0 ("Value") -1.0 ("Value") 0.0 ("Value")] -> w233
              tunnel: [255.0 ("Value") 1.0 ("Value") 5.0 ("Value")] -> w232
              tunnel: [128.0 ("Value") 0.0 ("Value") 0.0 ("Value")] -> w231
              tunnel: [64.0 ("Value") 0.5 ("Value") 1.0 ("Value")] -> w230
              frame "PWM" {
              }
              frame "Motor", Default {
              }
              frame "Analog Out" {
              }
            }
            n125 = property on="Motor" class="Clust (strict)"("Visible"=TRUE) -> ()  [unwired: 2 in, 2 out]
            n126 = property on="Value" class="Slide (strict)"("Value"=w231, "Scale.Minimum"=w233, "Scale.Maximum"=w232, "Scale.Increment"=w230) -> ()  [unwired: 2 in, 2 out]
            n127 = property on="On/Off" class="Bool (strict)"("Visible"=w235) -> ()  [unwired: 2 in, 2 out]
            n128 = property on="Test Slider" class="Slide (strict)"("Visible"=w235) -> ()  [unwired: 2 in, 2 out]
            n129 = property on="Test Ring" class="Ring (strict)"("Visible"=w235) -> ()  [unwired: 2 in, 2 out]
            n130 = property on="Rev/Fwd" class="Clust (strict)"("Visible"=w235) -> ()  [unwired: 2 in, 2 out]
          }
          frame "Servo" {
            w251 = FALSE ("Visible")
            n131 = call <vilib>:"NT Read Number.vi"("Name"=w253) -> ("Numeric"=w252:dbl)  [unwired: 9 in, 1 out]
            n132 = property on="Test Slider" class="Slide (strict)"("Visible"=TRUE, "Scale.Maximum"=170.0 ("Scale.Range:Maximum")) -> ()  [unwired: 2 in, 2 out]
            n133 = local write "Test Slider"(w252) -> ()
            n134 = property on="Motor" class="Clust (strict)"("Visible"=w251) -> ()  [unwired: 2 in, 2 out]
            n135 = property on="Rev/Fwd" class="Clust (strict)"("Visible"=w251) -> ()  [unwired: 2 in, 2 out]
            n136 = property on="On/Off" class="Bool (strict)"("Visible"=w251) -> ()  [unwired: 2 in, 2 out]
            n137 = property on="Test Ring" class="Ring (strict)"("Visible"=w251) -> ()  [unwired: 2 in, 2 out]
          }
          frame "Relay", "Solenoid" {
            w254 = FALSE ("Visible")
            n138 = property on="Motor" class="Clust (strict)"("Visible"=w254) -> ()  [unwired: 2 in, 2 out]
            n139 = property on="Test Slider" class="Slide (strict)"("Visible"=w254) -> ()  [unwired: 2 in, 2 out]
            n140 = Search and Replace String(input string=w255, search string="/Value  **", replace string="/Direction") -> (result string=w261:string)  [unwired: 5 in, 3 out]
            n141 = property on="Test Ring" class="Ring (strict)"("Visible"=w254) -> ()  [unwired: 2 in, 2 out]
            n142 = call <vilib>:"NT Read String.vi"("Name"=w261) -> ("String"=w259:string)  [unwired: 9 in, 1 out]
            n143 = Equal?(x="Both directions", y=w259) -> (x = y?=w257:bool)
            n144 = Not(x=w257) -> (.not. x?=w258:bool)
            n145 = property on="Rev/Fwd" class="Clust (strict)"("Visible"=w257) -> ()  [unwired: 2 in, 2 out]
            n146 = property on="On/Off" class="Bool (strict)"("Visible"=w258, "Caption.Text"=w256) -> ()  [unwired: 2 in, 2 out]
          }
          frame "Compressor", "Digital Out" {
            w264 = FALSE ("Visible")
            # "Get direction and finish"
            n147 = property on="Motor" class="Clust (strict)"("Visible"=w264) -> ()  [unwired: 2 in, 2 out]
            n148 = property on="Test Slider" class="Slide (strict)"("Visible"=w264) -> ()  [unwired: 2 in, 2 out]
            n149 = property on="Test Ring" class="Ring (strict)"("Visible"=w264) -> ()  [unwired: 2 in, 2 out]
            n150 = property on="On/Off" class="Bool (strict)"("Visible"=TRUE, "Caption.Text"=w265) -> ()  [unwired: 2 in, 2 out]
            n151 = property on="Rev/Fwd" class="Clust (strict)"("Visible"=FALSE) -> ()  [unwired: 2 in, 2 out]
          }
          frame "Camera" {
            n152 = call <vilib>:"Get Last Path Segment.vi"("String in"=w272) -> ("String out"=w273:string)  [unwired: 10 in]
            n153 = property on="On/Off" class="Bool (strict)"("Visible"=FALSE) -> ()  [unwired: 2 in, 2 out]
            n154 = property on="Motor" class="Clust (strict)"("Visible"=FALSE) -> ()  [unwired: 2 in, 2 out]
            n155 = property on="Rev/Fwd" class="Clust (strict)"("Visible"=FALSE) -> ()  [unwired: 2 in, 2 out]
            n156 = case shown="\"White Balance  **\"" w273 {
              tunnel: w272 -> [w279 w288 w297 w306 w315 _ w321]
              tunnel: w271 -> [w277 w285 w294 w303 w312 _ _]
              frame "Size  **" {
                n157 = Index Array(array=w277) -> (element=w276:cluster{string[]})  [unwired: 1 in]
                n158 = call <vilib>:"NT Read String.vi"("Name"=w279) -> ("String"=w278:string)  [unwired: 9 in, 1 out]
                n159 = Unbundle(w276) -> (w274:string[])
                n160 = Match First String(2:w274, 3:w278) -> (0:w275:i32)  [unwired: 1 out]
                n161 = property on="Test Ring" class="Ring (strict)"("Value"=w275, "Strings []"=w274) -> ()  [unwired: 2 in, 2 out]
                n162 = property on="Test Ring" class="Ring (strict)"("Visible"=TRUE) -> ()  [unwired: 2 in, 2 out]
                n163 = property on="Test Slider" class="Slide (strict)"("Visible"=FALSE) -> ()  [unwired: 2 in, 2 out]
              }
              frame "White Balance  **" {
                n164 = Index Array(array=w285, index=1) -> (element=w286:cluster{string[]})
                n165 = call <vilib>:"NT Read String.vi"("Name"=w288) -> ("String"=w287:string)  [unwired: 9 in, 1 out]
                n166 = Unbundle(w286) -> (w283:string[])
                n167 = Match First String(2:w283, 3:w287) -> (0:w282:i32)  [unwired: 1 out]
                n168 = property on="Test Ring" class="Ring (strict)"("Value"=w282, "Strings []"=w283) -> ()  [unwired: 2 in, 2 out]
                n169 = property on="Test Ring" class="Ring (strict)"("Visible"=TRUE) -> ()  [unwired: 2 in, 2 out]
                n170 = property on="Test Slider" class="Slide (strict)"("Visible"=FALSE) -> ()  [unwired: 2 in, 2 out]
              }
              frame "Exposure  **" {
                n171 = Index Array(array=w294, index=2) -> (element=w295:cluster{string[]})
                n172 = call <vilib>:"NT Read String.vi"("Name"=w297) -> ("String"=w296:string)  [unwired: 9 in, 1 out]
                n173 = Unbundle(w295) -> (w291:string[])
                n174 = Match First String(2:w291, 3:w296) -> (0:w292:i32)  [unwired: 1 out]
                n175 = property on="Test Ring" class="Ring (strict)"("Value"=w292, "Strings []"=w291) -> ()  [unwired: 2 in, 2 out]
                n176 = property on="Test Ring" class="Ring (strict)"("Visible"=TRUE) -> ()  [unwired: 2 in, 2 out]
                n177 = property on="Test Slider" class="Slide (strict)"("Visible"=FALSE) -> ()  [unwired: 2 in, 2 out]
              }
              frame "Exposure Priority  **" {
                n178 = Index Array(array=w303, index=3) -> (element=w304:cluster{string[]})
                n179 = call <vilib>:"NT Read String.vi"("Name"=w306) -> ("String"=w305:string)  [unwired: 9 in, 1 out]
                n180 = Unbundle(w304) -> (w300:string[])
                n181 = Match First String(2:w300, 3:w305) -> (0:w301:i32)  [unwired: 1 out]
                n182 = property on="Test Ring" class="Ring (strict)"("Value"=w301, "Strings []"=w300) -> ()  [unwired: 2 in, 2 out]
                n183 = property on="Test Ring" class="Ring (strict)"("Visible"=TRUE) -> ()  [unwired: 2 in, 2 out]
                n184 = property on="Test Slider" class="Slide (strict)"("Visible"=FALSE) -> ()  [unwired: 2 in, 2 out]
              }
              frame "Color Enable  **" {
                n185 = Index Array(array=w312, index=4) -> (element=w313:cluster{string[]})
                n186 = call <vilib>:"NT Read String.vi"("Name"=w315) -> ("String"=w314:string)  [unwired: 9 in, 1 out]
                n187 = Unbundle(w313) -> (w309:string[])
                n188 = Match First String(2:w309, 3:w314) -> (0:w310:i32)  [unwired: 1 out]
                n189 = property on="Test Ring" class="Ring (strict)"("Value"=w310, "Strings []"=w309) -> ()  [unwired: 2 in, 2 out]
                n190 = property on="Test Ring" class="Ring (strict)"("Visible"=TRUE) -> ()  [unwired: 2 in, 2 out]
                n191 = property on="Test Slider" class="Slide (strict)"("Visible"=FALSE) -> ()  [unwired: 2 in, 2 out]
              }
              frame Default {
                n192 = property on="Test Ring" class="Ring (strict)"("Visible"=FALSE) -> ()  [unwired: 2 in, 2 out]
                n193 = property on="Test Slider" class="Slide (strict)"("Visible"=FALSE) -> ()  [unwired: 2 in, 2 out]
              }
              frame "Brightness  **", "Color Level  **", "Compression  **", "FPS  **", "Sharpness  **" {
                n194 = call <vilib>:"NT Read Number.vi"("Name"=w321) -> ("Numeric"=w320:dbl)  [unwired: 9 in, 1 out]
                n195 = local write "Test Slider"(w320) -> ()
                n196 = property on="Test Slider" class="Slide (strict)"("Visible"=TRUE, "Scale.Maximum"=100.0 ("Scale.Range:Maximum")) -> ()  [unwired: 2 in, 2 out]
                n197 = property on="Test Ring" class="Ring (strict)"("Visible"=FALSE) -> ()  [unwired: 2 in, 2 out]
              }
            }
          }
        }
        n198 = property on="Progress" class="Clust (strict)"("Visible"=FALSE) -> ()  [unwired: 2 in, 2 out]
      }
      event "Test Name": Mouse Enter {
        # "Populate the ring with the list of tests"
        n199 = event-data() -> ()  [unwired: 1 in, 1 out]
        n200 = call <vilib>:"NT Read String Array.vi"("Name"="/TestMode/TestList") -> ("String Array"=w330:string[])  [unwired: 9 in, 1 out]
        n201 = Build Array (concatenate)("Select the test to run...", w330) -> (w329:string[])
        n202 = property on="Test Name" class="Ring (strict)"("Strings []"=w329) -> ()  [unwired: 2 in, 2 out]
      }
      event "Test Name": Value Change {
        w333 = FALSE ("Visible")
        # "Tell the robot the test name to run"
        n203 = event-data() -> ("NewVal"=w337:u16)  [unwired: 1 in]
        n204 = property on="Test Name" class="Ring (strict)"() -> ("Strings []"=w338:string[])  [unwired: 2 in, 2 out]
        n205 = local write "Progress"(T7 {"Test Progress"=0, "Test Progress Text"=""} ("Progress")) -> ()
        n206 = Index Array(array=w338, index=w337) -> (element=w336:string)
        n207 = call <vilib>:"NT Write String.vi"("String"=w336, "Name"="/TestMode/TestName") -> ()  [unwired: 9 in, 1 out]
        n208 = property on="Progress" class="Clust (strict)"("Visible"=TRUE) -> ()  [unwired: 2 in, 2 out]
        n209 = property on="Motor" class="Clust (strict)"("Visible"=w333) -> ()  [unwired: 2 in, 2 out]
        n210 = property on="Test Slider" class="Slide (strict)"("Visible"=w333) -> ()  [unwired: 2 in, 2 out]
        n211 = property on="On/Off" class="Bool (strict)"("Visible"=w333) -> ()  [unwired: 2 in, 2 out]
        n212 = property on="Rev/Fwd" class="Clust (strict)"("Visible"=w333) -> ()  [unwired: 2 in, 2 out]
        n213 = property on="Test Ring" class="Ring (strict)"("Visible"=w333) -> ()  [unwired: 2 in, 2 out]
      }
      event "Select Auto": Mouse Enter {
        # "Populate the combo box with the list of autonomous options"
        n214 = event-data() -> ()  [unwired: 1 in, 1 out]
        n215 = call <vilib>:"NT Read String Array.vi"("Name"="Auto List") -> ("String Array"=w340:string[])  [unwired: 9 in, 1 out]
        n216 = property on="Select Auto" class="CmbBox"("Strings[]"=w340) -> ()  [unwired: 2 in, 2 out]
      }
      event "Select Auto": Value Change {
        # "User modified the Auto Selection. Write to NT variable so robot knows."
        n217 = event-data() -> ("NewVal"=w344:string)  [unwired: 1 in]
        n218 = call <vilib>:"NT Write String.vi"("String"=w344, "Name"="Auto Selector") -> ()  [unwired: 9 in, 1 out]
      }
      event "Command Selection": Value Change {
        # "Get the params and show in table"
        n219 = event-data() -> ("NewVal"=w351:i32)  [unwired: 1 in]
        n220 = property on="Command Selection" class="MCListbox (strict)"() -> ("ItemNames"=w349:string[][])  [unwired: 2 in, 2 out]
        n221 = call <vilib>:"WPI_DashboardUpdate Command Params.vi"("NewVal"=w351, "Commands"=w349, "Param Tbl"=w350) -> ()  [unwired: 8 in, 1 out]
      }
      event "Execute Command": Value Change {
        # "Started one, Unique ID holds\nresponse"
        n222 = event-data() -> ()  [unwired: 1 in, 1 out]
        n223 = property on="Command Selection" class="MCListbox (strict)"() -> ("ItemNames"=w363:string[][])  [unwired: 2 in, 2 out]
        n224 = Index Array(array=w363, index (row)="Command Selection", index (col)=0) -> (element=w361:string)
        n225 = call <vilib>:"Invoke Commands.vi"("Command Params"="Command Params", "Function Name"=w361) -> ("Params"=w357:u8, "Started"=w356:bool)  [unwired: 7 in, 1 out]
        n226 = Array Subset(array="Command Params", length (row)=w357) -> (w358:string[][])  [unwired: 3 in]
        n227 = Select(t="Executing" ("Cmd Status"), s=w356, f="" ("Cmd Status")) -> (s? t:f=→"Cmd Status":string)
      }
      event "Command Selection": Double Click {
        n228 = event-data() -> ("Row"=w373:i32)  [unwired: 1 in]
        n229 = property on="Command Selection" class="MCListbox (strict)"() -> ("ItemNames"=w376:string[][])  [unwired: 2 in, 2 out]
        n230 = local read "Command Params"() -> (w371:string[][])
        n231 = Index Array(array=w376, index (row)=w373, index (col)=0) -> (element=w374:string)
        n232 = call <vilib>:"Invoke Commands.vi"("Command Params"=w371, "Function Name"=w374) -> ("Params"=w370:u8, "Started"=w365:bool)  [unwired: 7 in, 1 out]
        n233 = Array Subset(array=w371, length (row)=w370) -> (w369:string[][])  [unwired: 3 in]
        n234 = Select(t="Executing" ("Cmd Status"), s=w365, f="" ("Cmd Status")) -> (s? t:f=w366:string)
        n235 = local write "Cmd Status"(w366) -> ()
      }
      event "CheckList": Double Click {
        # "Shift clears all"
        # "Update symbols on the listbox"
        n236 = event-data() -> ("PlatMods.Shift"=w379:bool, "Row"=w381:i32)  [unwired: 1 in]
        n237 = case shown="True" w379 {
          tunnel: w381 -> [w385 _]
          tunnel: 1 -> [w384 _]
          frame False {
            n238 = property on="CheckList" class="LstBox (strict)"() -> ("Item Symbols"=w383:i32[])  [unwired: 2 in, 2 out]
            n239 = Replace Array Subset(array=w383, new element=w384, index=w385) -> (w382:i32[])
            n240 = property on="CheckList" class="LstBox (strict)"("Item Symbols"=w382) -> ()  [unwired: 2 in, 2 out]
          }
          frame True {
            w386 = 0 ("Top Row")
            n241 = property on="CheckList" class="LstBox (strict)"() -> ("Number of Rows"=w388:u32)  [unwired: 2 in, 2 out]
            n242 = Initialize Array(0, w388) -> (w387:i32[])
            n243 = property on="CheckList" class="LstBox (strict)"("Top Row"=w386, "Value"=w386, "Item Symbols"=w387) -> ()  [unwired: 2 in, 2 out]
          }
        }
      }
      event "CheckList": Key Down {
        # "Update symbols on the listbox\nLeft and right keys check and uncheck"
        n244 = event-data() -> ("VKey"=w393:T22)  [unwired: 1 in]
        n245 = case shown="\"Left\", \"Right\"" w393 {
          selector: w393 -> [w398 _]
          tunnel: eventvkey."Left" ("VKey") -> [w396 _]
          frame "Left", "Right" {
            n246 = Equal?(x=w396, y=w398) -> (x = y?=w397:bool)
            n247 = Select(t=0, s=w397, f=1) -> (s? t:f=w399:i32)
            n248 = property on="CheckList" class="LstBox (strict)"() -> ("Item Symbols"=w402:i32[])  [unwired: 2 in, 2 out]
            n249 = Replace Array Subset(array=w402, new element=w399, index="CheckList") -> (w401:i32[])
            n250 = property on="CheckList" class="LstBox (strict)"("Item Symbols"=w401) -> ()  [unwired: 2 in, 2 out]
          }
          frame Default {
          }
        }
      }
      event "DB Camera Config": Value Change {
        # "Show or hide the cluster of controls, store in ini file"
        n251 = event-data() -> ("NewVal"=w407:bool)  [unwired: 1 in]
        n252 = case shown="False" w407 {
          tunnel: w406 -> [w416 _]
          tunnel: [w409 w427] -> w405
          tunnel: w404 -> [w408 w427]
          frame False {
            w423 = "Camera"
            w426 = FALSE ("Visible")
            n253 = local read "Camera Settings"() -> (w415:T2)
            n254 = Index Array(array=w416) -> (element=w419:cluster{string[]})  [unwired: 1 in]
            n255 = Unbundle(w415) -> ("Frame Rate"=w414:i32, "Compression"=w413:i32, "Size"=w417:u16)
            n256 = Unbundle(w419) -> (w418:string[])
            n257 = Index Array(array=w418, index=w417) -> (element=w412:string)
            n258 = call-poly <vilib>:"Write Key.vi"("section"=w423, "value"=w412, "key"="Size", "refnum"=w408) -> ("refnum out"=w425:T20)  [unwired: 2 in, 5 out]
            n259 = call-poly <vilib>:"Write Key.vi"("section"=w423, "value"=w414, "key"="FrameRate", "refnum"=w425) -> ("refnum out"=w424:T20)  [unwired: 1 in, 6 out]
            n260 = property on="Camera Settings" class="Clust (strict)"("Visible"=w426) -> ()  [unwired: 2 in, 2 out]
            n261 = local write "DB Camera Config"(w426) -> ()
            n262 = call-poly <vilib>:"Write Key.vi"("section"=w423, "value"=w413, "key"="Compression", "refnum"=w424) -> ("refnum out"=w410:T20)  [unwired: 1 in, 6 out]
            n263 = call <vilib>:"Close Config Data.vi"("refnum"=w410) -> ("file path"=w411:path)  [unwired: 2 in, 8 out]
            n264 = call <vilib>:"Open Config Data.vi"("configuration file path"=w411) -> ("refnum"=w409:T20)  [unwired: 8 in, 2 out]
          }
          frame True {
            n265 = property on="Camera Settings" class="Clust (strict)"("Visible"=TRUE) -> ()  [unwired: 2 in, 2 out]
          }
        }
      }
      event "Camera Settings": Value Change {
        # "Update summary string when any elements of DB camera change"
        n266 = event-data() -> ("NewVal"=w441:T2)  [unwired: 1 in]
        n267 = Index Array(array=w437) -> (element=w436:cluster{string[]})  [unwired: 1 in]
        n268 = Unbundle(w441) -> ("Frame Rate"=w432:i32, "Compression"=w431:i32, "Size"=w434:u16)
        n269 = Unbundle(w436) -> (w435:string[])
        n270 = Index Array(array=w435, index=w434) -> (element=w433:string)
        n271 = Format Into String(format string="%s   %dfps   %d%%", w433, w432, w431) -> (resulting string=w438:string)  [unwired: 2 in, 1 out]
        n272 = Build Array(w438) -> (w439:string[])
        n273 = property on="DB Camera Config" class="Bool (strict)"("Strings [4]"=w439) -> ()  [unwired: 2 in, 2 out]
      }
      event "Motor.Enable": Value Change {
        # "When the test mode otor enable helper is set, update that\ntree row item's value"
        n274 = event-data() -> ("NewVal"=w448:bool)  [unwired: 1 in]
        n275 = Unbundle("Motor") -> ("Value"=w447:dbl)  [unwired: 1 out]
        n276 = Select(t=w447, s=w448, f=0.0) -> (s? t:f=w445:dbl)
        n277 = call <vilib>:"NT Write Number.vi"("Numeric"=w445, "Name"=w444) -> ()  [unwired: 9 in, 1 out]
      }
      event "Test Slider": Value Change {
        # "When the test mode slider helper is set, update that\ntree row item's value"
        n278 = event-data() -> ("NewVal"=w452:dbl)  [unwired: 1 in]
        n279 = call <vilib>:"NT Write Number.vi"("Numeric"=w452, "Name"=w453) -> ()  [unwired: 9 in, 1 out]
      }
      event "On/Off": Value Change {
        # "When the test mode on/off helper value is set, update that\ntree row item's value"
        n280 = event-data() -> ("NewVal"=w458:bool)  [unwired: 1 in]
        n281 = Boolean To (0,1)(Boolean=w458) -> (0, 1=w457:i16)
        n282 = call <vilib>:"NT Write Number.vi"("Numeric"=w457, "Name"=w456) -> ()  [unwired: 9 in, 1 out]
      }
      event "Rev/Fwd": Value Change {
        # "When the test mode helper value for relays is set, update that\ntree row item's value"
        n283 = event-data() -> ("NewVal.Forward"=w467:bool, "NewVal.Reverse"=w466:bool)  [unwired: 1 in]
        n284 = Boolean To (0,1)(Boolean=w467) -> (0, 1=w463:i16)
        n285 = Boolean To (0,1)(Boolean=w466) -> (0, 1=w465:i16)
        n286 = Negate(x=w465) -> (-x=w464:i16)
        n287 = Add(x=w463, y=w464) -> (x+y=w462:i16)
        n288 = call <vilib>:"NT Write Number.vi"("Numeric"=w462, "Name"=w461) -> ()  [unwired: 9 in, 1 out]
      }
      event "Test Ring": Value Change {
        # "When a test mode helper value is selected from the ring,\nset the tree item's variable to the string value"
        n289 = event-data() -> ("NewVal"=w472:u16)  [unwired: 1 in]
        n290 = property on="Test Ring" class="Ring (strict)"() -> ("Strings []"=w473:string[])  [unwired: 2 in, 2 out]
        n291 = Index Array(array=w473, index=w472) -> (element=w471:string)
        n292 = call <vilib>:"NT Write String.vi"("String"=w471, "Name"=w470) -> ()  [unwired: 9 in, 1 out]
      }
      event "Rec Mode": Value Change {
        # "Update globals for recording mode and path to read log from.\nClear when logging and let NetworkTables set path for vision to\nuse."
        n293 = event-data() -> ("NewVal"=w485:enum32{"Stop", "Record", "Playback"})  [unwired: 1 in]
        n294 = global write "WPI_DashboardLogging Global.vi" "Logging Filename"(path "") -> ()
        n295 = global write "WPI_DashboardLogging Global.vi" "Recording"(w485) -> ()
        n296 = case shown="\"Playback\"" w485 {
          tunnel: w484 -> [_ w487 w496]
          tunnel: [_ _ w495] -> w481
          tunnel: [_ _ w494] -> _
          tunnel: w479 -> [_ _ w492]
          tunnel: cluster{i32, i32} {-250, 170} -> [_ _ w491]
          tunnel: [_ _ T23 {"Image Size"=TRUE, "Image Type"=TRUE, "Pixel Value"=TRUE, "ROI Information"=TRUE, "Zoom Factor"=FALSE} ("Image Information Shown:All Elements")] -> w477
          tunnel: [_ _ TRUE ("Zoom Factor")] -> w476
          tunnel: w475 -> [_ _ w488]
          frame Default {
          }
          frame "Stop", "Record" {
            # "Place Window too"
            n297 = invoke class="VI" method="FP.Close"(reference=w487) -> (reference out=w486:refnum<vi>)  [unwired: 2 in, 2 out]
            n298 = invoke class="VI" method="Abort VI"(reference=w486) -> ()  [unwired: 2 in, 3 out]
          }
          frame "Playback" {
            n299 = call "Open Playback Panel.vi"("Offset"=w491, "DB VI Ref"=w492, "Playback in"=w496) -> ("Playback out"=w493:refnum<vi>)  [unwired: 8 in]
            n300 = register-events(w493, w488) -> (reference out=w495:refnum<event-registration>, error out=w494:errorcluster)  [unwired: 2 in]
          }
        }
        n301 = property on="Camera Image" class="ImageControl"("Image Information Shown"=w477, "Image Information Visible"=w476) -> ()  [unwired: 2 in, 2 out]
        n302 = call <vilib>:"WPI_DashboardNT Log FieldName Cache.vi"("Operation"=enum16{"Lookup/Add", "Index", "Clear"}."Clear") -> ()  [unwired: 8 in, 3 out]
      }
      event Panel Close {
        w498 = enum32{"Stop", "Record", "Playback"}."Stop" ("Rec Mode")
        # "Playback window has been closed, abort"
        n303 = event-data() -> ()  [unwired: 1 in, 4 out]
        n304 = local write "Rec Mode"(w498) -> ()
        n305 = global write "WPI_DashboardLogging Global.vi" "Recording"(w498) -> ()
      }
      event Panel Close {
        # "Abort playback window and ourself"
        n306 = event-data() -> ()  [unwired: 1 in, 4 out]
        n307 = invoke class="VI" method="FP.Close"(reference=w504) -> (reference out=w503:refnum<vi>)  [unwired: 2 in, 2 out]
        n308 = invoke class="VI" method="Abort VI"(reference=w503) -> (error out=w502:errorcluster)  [unwired: 2 in, 2 out]
        n309 = invoke class="VI" method="Abort VI"(error in=w502) -> ()  [unwired: 2 in, 3 out]
      }
      event User Event {
        n310 = event-data() -> ("IDs"=w512:cluster{"RPC field ID":u16, "Unique ID":u16}, "String"=w511:string)  [unwired: 1 in]
        n311 = Bundle("IDs"=w512, "String"=w511) -> (w510:T9)  [unwired: 1 in]
        n312 = call <vilib>:"Retrieve RPC Response.vi"("RPC Response"=w510) -> ("Output"=w507:string[][])  [unwired: 10 in]
        n313 = Build Array (concatenate)(w505, w507) -> (w506:string[][])
        n314 = local write "Command Params"(w506) -> ()
        n315 = local write "Cmd Status"("" ("Cmd Status")) -> ()
      }
      event "Vision": Value Change {
        # "Enable/Disable Compression slider.\nHW USB is hard-coded into the camera"
        n316 = event-data() -> ("NewVal"=w519:u16)  [unwired: 1 in]
        n317 = Equal?(x=w519, y=u32 2 ("milliseconds to wait")) -> (x = y?=w517:bool)
        n318 = Select(t=T24."Disabled and Grayed Out" ("Disabled"), s=w517, f=T24."Enabled" ("Disabled")) -> (s? t:f=w514:T24)
        n319 = property on="Compression" class="Slide (strict)"("DisabledEnum"=w514) -> ()  [unwired: 2 in, 2 out]
      }
      event "Tree": Double Click {
        n320 = event-data() -> ("PlatMods"=w524:T27, "Tag"=w523:string)  [unwired: 1 in]
        n321 = Unbundle(w524) -> ("Shift"=w522:bool)  [unwired: 4 out]
        n322 = Not(x=w522) -> (.not. x?=w521:bool)
        n323 = call <vilib>:"NT Update Persistence.vi"("Persistence"=w521, "Name"=w523) -> ()  [unwired: 9 in, 1 out]
      }
    }
  }
  n324 = while {
    tunnel: w47 -> [w528]
    i -> [w531]
    stop <- FALSE stop-if-true
    n325 = Wait (ms)(milliseconds to wait=u32 100) -> ()  [unwired: 1 out]
    n326 = case shown="\"Playback\"" "Rec Mode" {
      tunnel: w531 -> [_ _ w546]
      tunnel: [u32 2829099 ("Base Color") u32 11141120 ("Target Color") w535] -> w527
      frame "Stop", Default {
        # "Reset the color, extra updates don't cost much"
      }
      frame "Record" {
      }
      frame "Playback" {
        # "Playback"
        n327 = Quotient & Remainder(x=w546, y=u32 50 ("milliseconds to wait")) -> (x-y*floor(x/y)=w542:u32)  [unwired: 1 out]
        n328 = Divide(x=w542, y=u32 50 ("milliseconds to wait")) -> (x/y=w539:dbl)
        n329 = Multiply(x=6.283185307179586, y=w539) -> (x*y=w544:dbl)
        n330 = Sine(x=w544) -> (sin(x)=w543:dbl)
        n331 = Absolute Value(x=w543) -> (abs(x)=w536:dbl)
        n332 = call "Interpolate RGB Color.vi"("Proportion"=w536, "Target Color"=u32 30976, "Base Color"=u32 2829099) -> ("Result Color"=w535:u32)  [unwired: 8 in]
      }
    }
    n333 = property class="Pane"(reference=w528, "PaneColor"=w527) -> ()  [unwired: 1 in, 2 out]
  }
  n334 = local write "Dashboard Tab"(T1."Drive" ("Dashboard Tab")) -> ()
  n335 = property on="On/Off" class="Bool (strict)"("Visible"=w15) -> ()  [unwired: 2 in, 2 out]
  n336 = property on="Motor" class="Clust (strict)"("Visible"=w15) -> ()  [unwired: 2 in, 2 out]
  n337 = property on="Progress" class="Clust (strict)"("Visible"=w15) -> ()  [unwired: 2 in, 2 out]
  n338 = property on="Test Ring" class="Ring (strict)"("Visible"=w15) -> ()  [unwired: 2 in, 2 out]
  n339 = property on="Rev/Fwd" class="Clust (strict)"("Visible"=w15) -> ()  [unwired: 2 in, 2 out]
  n340 = property on="Camera Settings" class="Clust (strict)"("Visible"=w15) -> ()  [unwired: 2 in, 2 out]
  n341 = while {
    tunnel: u16 1741 ("timeout ms (25000)") -> [w548]
    stop <- FALSE stop-if-true
    n342 = TCP Create Listener(10:w548) -> (0:w547:errorcluster, 3:w549:refnum<k5>)  [unwired: 4 in, 1 out]
    n343 = case shown="No Error" w547 {
      selector: w547 -> [w551 _]
      tunnel: w549 -> [w552 _]
      frame No Error {
        n344 = while {
          tunnel: w552 -> [w555]
          tunnel: w551 -> [w554]
          stop <- FALSE stop-if-true
          n345 = TCP Wait On Listener(8:w554, 11:w555) -> (0:w556:errorcluster, 4:w557:refnum<k5>)  [unwired: 2 in, 3 out]
          n346 = local write "TCP"(w557) -> ()
          n347 = case shown="No Error" w556 {
            frame No Error {
            }
            frame Error {
              n348 = Wait (ms)(milliseconds to wait=u32 1000) -> ()  [unwired: 1 out]
            }
          }
        }
      }
      frame Error {
        n349 = Wait (ms)(milliseconds to wait=u32 1000) -> ()  [unwired: 1 out]
      }
    }
  }
  n350 = local write "DB Camera Config"(w15) -> ()
  n351 = local write "Command Params"(string[][] [] ("Command Params")) -> ()
  n352 = global write "WPI_DashboardLogging Global.vi" "Recording"(w41) -> ()
  n353 = local write "Command Selection"(u16 0 ("milliseconds to wait")) -> ()
  n354 = local write "Rec Mode"(w41) -> ()
